vi "Ping.vi"(8 "error in (no error)":errorcluster, 11 "GH2 in":refnum<class "GH2.lvclass">) -> (0 "error out":errorcluster, 3 "GH2 out":refnum<class "GH2.lvclass">)   [LabVIEW 2026, in "GH2.lvclass"]
uses:
  GH2.lvclass
  GH2.lvclass/GH2.ctl
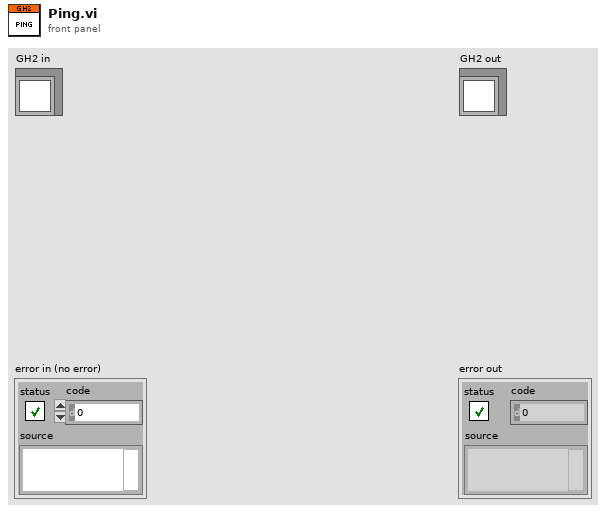
[diagram p1: front panel]
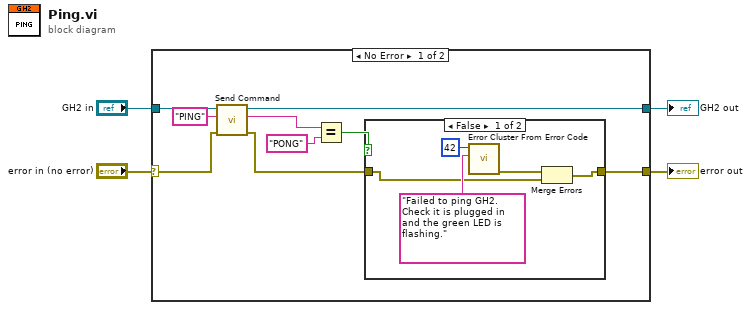
[diagram p0: block diagram]
diagram:
  n1 = case shown="No Error" "error in (no error)" {
    selector: "error in (no error)" -> [w11 w21]
    tunnel: [w5 w21] -> w3
    tunnel: [w12 w20] -> w1
    tunnel: "GH2 in" -> [w13 w20]
    frame No Error {
      n2 = call "Send Command.vi"("error in (no error)"=w11, "command"="PING", "GH2 in"=w13) -> ("error out"=w6:errorcluster, "response"=w9:string, "GH2 out"=w12:refnum<class "GH2.lvclass">)  [unwired: 6 in]
      n3 = Equal?(x=w9, y="PONG") -> (x = y?=w7:bool)
      n4 = case shown="False" w7 {
        tunnel: w6 -> [w16 w19]
        tunnel: [w14 w19] -> w5
        frame False {
          n5 = call <vilib>:"Error Cluster From Error Code.vi"("error message (\"\")"="Failed to ping GH2. Check it is plugged in and the green LED is flashing." ("error message (\"\")"), "error code (0)"=42) -> ("error out"=w15:errorcluster)  [unwired: 7 in]
          n6 = Merge Errors(w15, w16) -> (w14:errorcluster)
        }
        frame True {
        }
      }
    }
    frame Error {
    }
  }
  "error out" <- w3
  "GH2 out" <- w1
